vi "Read Size.vi"() -> (0 "bytes to read":i32)   [LabVIEW 2015, in "MJPEG Reader.lvclass"]
uses:
  MJPEG Reader.lvclass
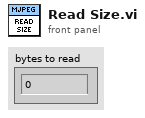
[diagram p1: front panel]
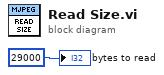
[diagram p0: block diagram]
diagram:
  "bytes to read" <- 29000 ("bytes to read")
